vi "Disconnect from Slave.vi"(8 "error in":errorcluster, 11 "TCP master in":refnum<class "SMSD Master.lvclass">) -> (0 "error out":errorcluster, 3 "TCP master out":refnum<class "SMSD Master.lvclass">)   [LabVIEW 2021, in "SMSD Master.lvclass"]
doc: "Closes the TCP connection stored in the class."
uses:
  SMSD Master.lvclass
  SMSD Master.lvclass/SMSD Master.ctl
  Transmission Data Unit/SMSD/SMSD ADU.lvclass/SMSD ADU.ctl
  Transmission Data Unit/SMSD/SMSD ADU.lvclass
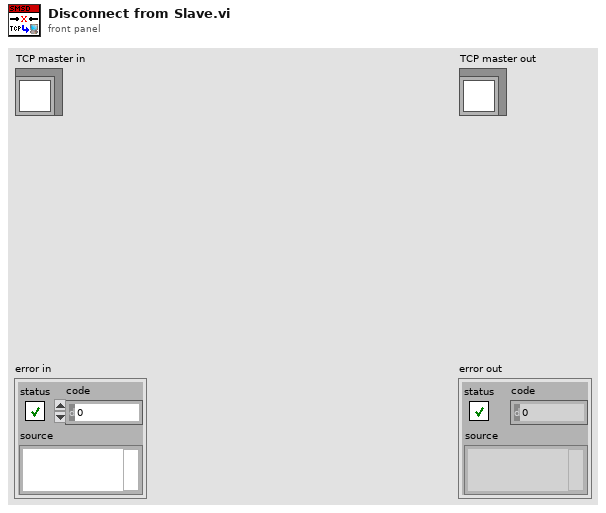
[diagram p1: front panel]
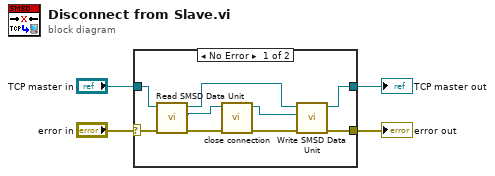
[diagram p0: block diagram]
diagram:
  n1 = case shown="No Error" "error in" {
    selector: "error in" -> [w9 w15]
    tunnel: "TCP master in" -> [w12 w14]
    tunnel: [w11 w15] -> w3
    tunnel: [w10 w14] -> w2
    frame No Error {
      n2 = call "Read SMSD Data Unit.vi"("error in (no error)"=w9, "SMSD Master in"=w12) -> ("error out"=w8:errorcluster, "IP Data Unit"=w6:refnum<class "SMSD ADU.lvclass">, "SMSD Master out"=w13:refnum<class "SMSD Master.lvclass">)  [unwired: 7 in]
      n3 = call "close connection.vi"("error in"=w8, "TCP master in"=w6) -> ("error out"=w7:errorcluster, "TCP master out"=w5:refnum<class "SMSD ADU.lvclass">)  [unwired: 8 in]
      n4 = call "Write SMSD Data Unit.vi"("error in (no error)"=w7, "IP Data Unit"=w5, "SMSD Master in"=w13) -> ("error out"=w11:errorcluster, "SMSD Master out"=w10:refnum<class "SMSD Master.lvclass">)  [unwired: 7 in]
    }
    frame Error {
    }
  }
  "error out" <- w3
  "TCP master out" <- w2
